vi "LoadFPObjectConfiguration.vi"(0 "FP Name":string, 2 "Objects":string[](array[string])) -> (14 "All Objects Configured":bool, 16 "Objects Configurations":T1[](array[typedef]))   [LabVIEW 2014, in "FrontPanelPublisher.lvlib" / "WebFrontPanel.lvclass"]
uses:
  WebFrontPanel.lvclass
  Controls/FPObjectConfiguration.ctl
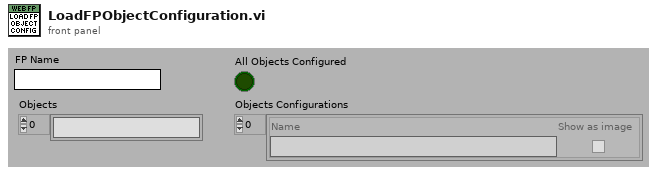
[diagram p1: front panel]
types:
  T1 = typedef "FrontPanelPublisher.lvlib/WebFrontPanel.lvclass/FPObjectConfiguration.ctl" = cluster{"Name":string, "Show as image":bool}
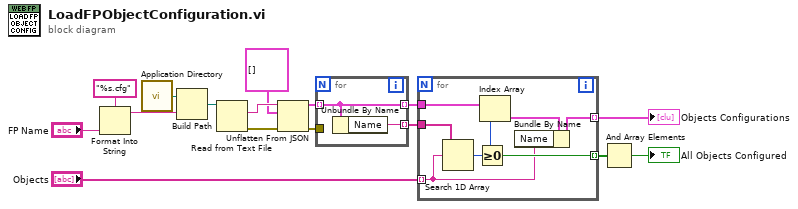
[diagram p0: block diagram]
diagram:
  n1 = Format Into String(format string="%s.cfg", "FP Name") -> (resulting string=w13:string)  [unwired: 2 in, 1 out]
  n2 = call <vilib>:"Application Directory.vi"() -> ("Application Directory"=w15:path)
  n3 = Build Path(base path=w15, name or relative path=w13) -> (appended path=w12:path)
  n4 = Read from Text File(file (use dialog)=w12) -> (text=w11:string, error out=w9:errorcluster)  [unwired: 3 in, 2 out]
  n5 = Unflatten From JSON(JSON string=w11, type and defaults=T1[] [], error in (no error)=w9) -> (value=w8:T1[], error out=w7:errorcluster)  [unwired: 4 in]
  n6 = for {
    tunnel: w8 -> [w17] mode=indexing
    tunnel: w7 -> [_]
    tunnel: [w18] -> w5 mode=indexing
    tunnel: [w17] -> w4 mode=indexing
    n7 = Unbundle By Name(w17) -> ("Name"=w18:string)
  }
  n8 = for {
    tunnel: "Objects" -> [w19] mode=indexing
    tunnel: [w20] -> w3 mode=indexing
    tunnel: w5 -> [w25]
    tunnel: w4 -> [w24]
    tunnel: [w22] -> w2 mode=indexing
    n9 = Search 1D Array(1D array=w25, element=w19) -> (index of element=w23:i32)  [unwired: 1 in]
    n10 = Greater Or Equal To 0?(x=w23) -> (x >= 0?=w22:bool)
    n11 = Index Array(array=w24, index=w23) -> (element=w21:T1)
    n12 = Bundle By Name(cluster=w21, "Name"=w19) -> (w20:T1)
  }
  "Objects Configurations" <- w3
  n13 = And Array Elements(Boolean array=w2) -> (logical AND=→"All Objects Configured":bool)
